vi "Start log_path.vi"(8 "error in (no error)":errorcluster, 10 "Data type":string="instrinsic", 11 "elative path":string="INTRINSIC") -> (0 "error out":errorcluster, 1 "Logging":bool, 3 "Path":path)   [LabVIEW 2016]
uses:
  <vilib>/Utility/sysdir.llb/System Directory Type.ctl
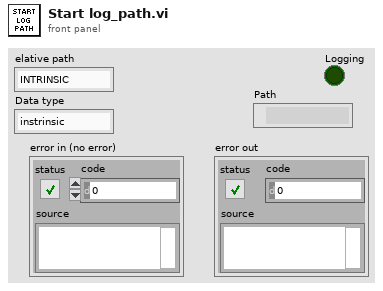
[diagram p1: front panel]
types:
  T1 = typedef "System Directory Type.ctl" = i32
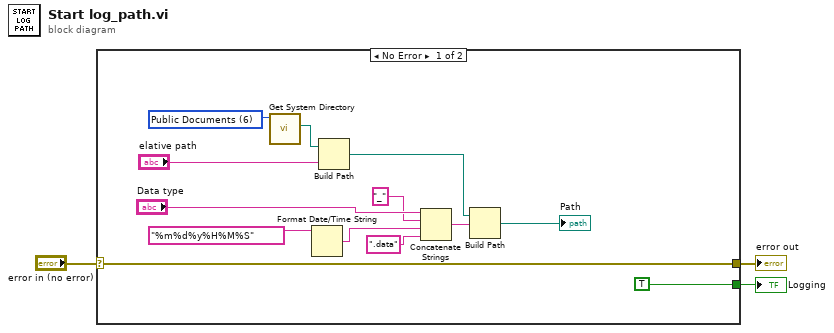
[diagram p0: block diagram]
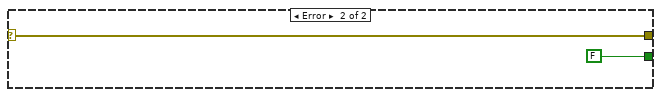
[diagram p2: hidden frame]
diagram:
  n1 = case shown="No Error" "error in (no error)" {
    selector: "error in (no error)" -> [w5 w18]
    tunnel: [w5 w18] -> w3
    tunnel: [TRUE FALSE] -> w1
    frame No Error {
      w12 = T1 6 items=["User Home"=0, "User Desktop"=1, "User Documents"=2, "User Application Data"=3, "User Preferences"=4, "User Temporary"=5, "Public Documents"=6, "Public Application Data"=7, "Public Preferences"=8, "Public Cache"=13, "System Core Libraries"=9, "System Installed Libraries"=10, "Application Files"=11, "Boot Volume Root"=12] ("system directory type")
      n2 = call <vilib>:"Get System Directory.vi"("system directory type"=w12) -> ("system directory"=w14:path)  [unwired: 10 in]
      n3 = Format Date/Time String(time format string (%c)="%m%d%y%H%M%S") -> (date/time string=w8:string)  [unwired: 2 in]
      n4 = Build Path(base path=w14, name or relative path="elative path") -> (appended path=w6:path)
      n5 = Concatenate Strings("Data type", "_", w8, ".data") -> (w11:string)
      n6 = Build Path(base path=w6, name or relative path=w11) -> (appended path=→"Path":path)
    }
    frame Error {
    }
  }
  "error out" <- w3
  "Logging" <- w1
